vi "AlliGator Get FLI Image Folder Metadata.vi"(8 "error in (no error)":errorcluster, 11 "Image Folder in":path) -> (0 "error out":errorcluster, 1 "Metadata":T1 {"Date" format="%<%x %.3X>T"}, 2 "Metadata String":string, 3 "Image Folder out":path)   [LabVIEW 2021, in "AlliGator Files.lvlib"]
doc: "Tries different ways to extract FLI dataset metadata corresponding to different vendor formats."
uses:
  AlliGator Files.lvlib
  AlliGator RecSettings Metadata.ctl
panel:
  # "see the AlliGator License on the block diagram (Ctrl+E or Window:Show Block Diagram)"
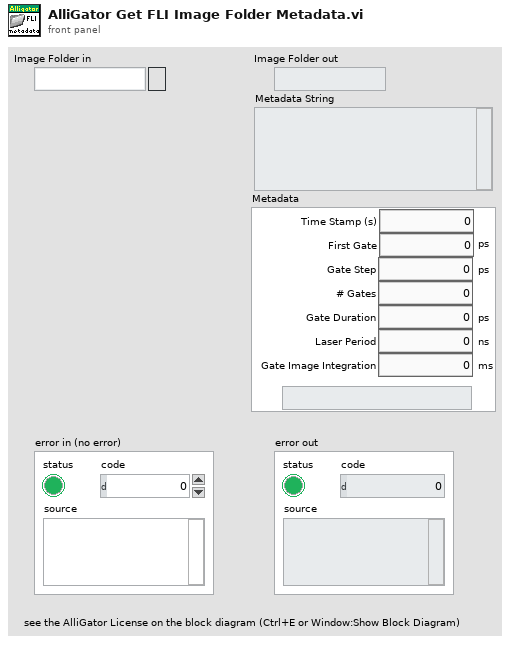
[diagram p1: front panel]
types:
  T1 = typedef "AlliGator Files.lvlib/AlliGator RecSettings Metadata.ctl" = cluster{"Time Stamp (s)":dbl, "First Gate":dbl[unit], "Gate Step":dbl[unit], "# Gates":i32, "Gate Duration":dbl[unit], "Laser Period":dbl[unit], "Gate Image Integration":dbl[unit], "Date":timestamp}
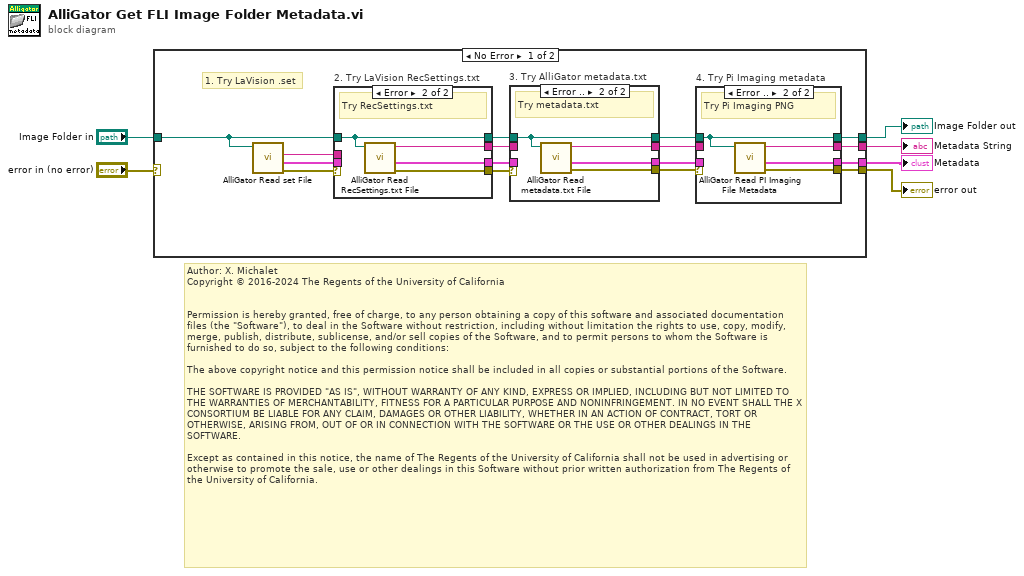
[diagram p0: block diagram]
diagram:
  # "Author: X. Michalet\nCopyright © 2016-2024 The Regents of the University of California\n \n\nPermission is hereby granted, free of charge, to any person obtaining a copy of this software and associated documentation files (the \"Software\"), to deal in the Software without restriction, including without limitation the rights to use, copy, modify, merge, publish, distribute, sublicense, and/or sell copies of the Software, and to permit persons to whom the Software is furnished to do so, subject to the following conditions:\n\nThe above copyright notice and this permission notice shall be included in all copies or substantial portions of the Software.\n\nTHE SOFTWARE IS PROVIDED \"AS IS\", WITHOUT WARRANTY OF ANY KIND, EXPRESS OR IMPLIED, INCLUDING BUT NOT LIMITED TO THE WARRANTIES OF MERCHANTABILITY, FITNESS FOR A PARTICULAR PURPOSE AND NONINFRINGEMENT. IN NO EVENT SHALL THE X CONSORTIUM BE LIABLE FOR ANY CLAIM, DAMAGES OR OTHER LIABILITY, WHETHER IN AN ACTION OF CONTRACT, TORT OR OTHERWISE, ARISING FROM, OUT OF OR IN CONNECTION WITH THE SOFTWARE OR THE USE OR OTHER DEALINGS IN THE SOFTWARE.\n\nExcept as contained in this notice, the name of The Regents of the University of California shall not be used in advertising or otherwise to promote the sale, use or other dealings in this Software without prior written authorization from The Regents of the University of California."
  n1 = case shown="No Error" "error in (no error)" {
    selector: "error in (no error)" -> [_ w48]
    tunnel: [w21 w48] -> w5
    tunnel: [w20 _] -> w4
    tunnel: [w19 _] -> w3
    tunnel: [w18 w47] -> w2
    tunnel: "Image Folder in" -> [w22 w47]
    frame No Error {
      # "1. Try LaVision .set"
      n2 = call "AlliGator Read set File.vi"("Image Folder Path"=w22) -> ("Error Out"=w13:errorcluster, "Metadata"=w7:T1, "File Info String"=w12:string)  [unwired: 6 in, 2 out]
      n3 = case "2. Try LaVision RecSettings.txt" shown="Error" w13 {
        selector: w13 -> [w41 _]
        tunnel: w12 -> [w42 _]
        tunnel: [w42 w46] -> w8
        tunnel: w22 -> [w40 w43]
        tunnel: [w41 w45] -> w11
        tunnel: [w39 w44] -> w9
        tunnel: [w40 w43] -> w10
        tunnel: w7 -> [w39 _]
        frame No Error {
        }
        frame Error {
          # "Try RecSettings.txt"
          n4 = call "AlliGator Read RecSettings.txt File.vi"("Folder Path"=w43) -> ("Error Out"=w45:errorcluster, "Metadata"=w44:T1, "Settings String"=w46:string)  [unwired: 8 in]
        }
      }
      n5 = case "3. Try AlliGator metadata.txt" shown="Error .." w11 {
        selector: w11 -> [w31 _]
        tunnel: w10 -> [w32 w35]
        tunnel: w9 -> [w34 _]
        tunnel: [w34 w37] -> w17
        tunnel: w8 -> [w33 _]
        tunnel: [w33 w38] -> w16
        tunnel: [w31 w36] -> w14
        tunnel: [w32 w35] -> w15
        frame No Error {
        }
        frame Error {
          # "Try metadata.txt"
          n6 = call "AlliGator Read metadata.txt File.vi"("Folder Path"=w35) -> ("Error Out"=w36:errorcluster, "Metadata"=w37:T1, "Settings String"=w38:string)  [unwired: 7 in, 1 out]
        }
      }
      n7 = case "4. Try Pi Imaging metadata" shown="Error .." w14 {
        selector: w14 -> [w23 _]
        tunnel: w15 -> [w26 w30]
        tunnel: w16 -> [w25 _]
        tunnel: w17 -> [w24 _]
        tunnel: [w26 w30] -> w18
        tunnel: [w25 w29] -> w19
        tunnel: [w24 w27] -> w20
        tunnel: [w23 w28] -> w21
        frame No Error {
        }
        frame Error {
          # "Try Pi Imaging PNG"
          n8 = call "AlliGator Read PI Imaging File Metadata.vi"("Image Folder"=w30) -> ("error out"=w28:errorcluster, "Metadata"=w27:T1, "Metadata String"=w29:string)  [unwired: 6 in, 2 out]
        }
      }
    }
    frame Error {
    }
  }
  "error out" <- w5
  "Metadata" <- w4
  "Metadata String" <- w3
  "Image Folder out" <- w2
